vi "dfd_Bilinear Warping of f.vi"(1 "f":dbl) -> (0 "prewarped f":dbl)   [LabVIEW 2017, in "NI_DigFilter_Design.lvlib"]
uses:
  <vilib>/addons/Digital Filter Design/NI_DigFilter_Design.lvlib
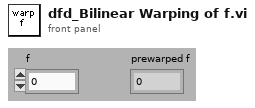
[diagram p1: front panel]
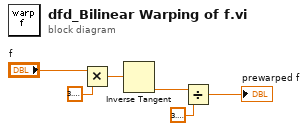
[diagram p0: block diagram]
diagram:
  n1 = Multiply(x="f", y=3.141592653589793) -> (x*y=w6:dbl)
  n2 = Inverse Tangent(1:w6) -> (0:w3:dbl)
  n3 = Divide(x=w3, y=3.141592653589793) -> (x/y=→"prewarped f":dbl)
